vi "Set OVP.vi"(8 "error in":errorcluster, 10 "OVP Level (0 V)":dbl min=0.0 max=32.0 step=0.1 format="%#_13g", 11 "Modbus instance in":refnum<class "Modbus API.lvclass">) -> (0 "error out":errorcluster, 3 "Modbus instance out":refnum<class "Modbus API.lvclass">)   [LabVIEW 2025, in "Hanmatek HM310T.lvlib"]
uses:
  <vilib>/NI/Modbus Library/API/Modbus API.lvclass
  <instrlib>/Hanmatek HM310T/Hanmatek HM310T.lvlib
  705d687a-c619-40f2-8314-2aba8980c0aa.vi
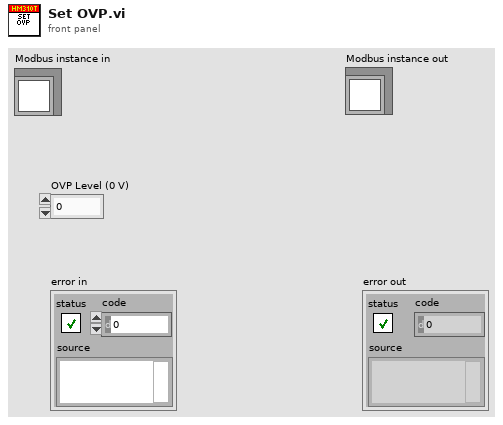
[diagram p1: front panel]
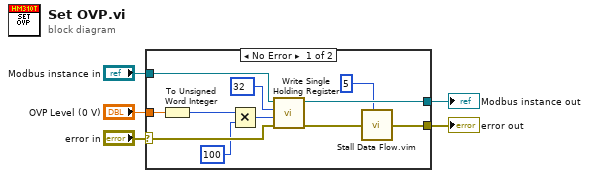
[diagram p0: block diagram]
diagram:
  n1 = case shown="No Error" "error in" {
    selector: "error in" -> [w15 w18]
    tunnel: [w7 w18] -> w4
    tunnel: [w14 w17] -> w2
    tunnel: "OVP Level (0 V)" -> [w11 _]
    tunnel: "Modbus instance in" -> [w9 w17]
    frame No Error {
      n2 = To Unsigned Word Integer(number=w11) -> (unsigned 16bit integer=w10:u16)
      n3 = Multiply(x=w10, y=u16 100) -> (x*y=w12:u16)
      n4 = call-dynamic "Write Single Holding Register.vi"("error in"=w15, "register to write"=w12, "address"=u16 32 ("Quantity of words (1)"), "Modbus instance in"=w9) -> ("error out"=w8:errorcluster, "Modbus instance out"=w14:refnum<class "Modbus API.lvclass">)  [unwired: 6 in]
      n5 = call "Stall Data Flow.vim"("value in"=w8, "milliseconds to wait"=u32 5) -> ("value out"=w7:errorcluster)  [unwired: 1 out]
    }
    frame Error {
    }
  }
  "error out" <- w4
  "Modbus instance out" <- w2
